vi "ReadJSONoverTCP.vi"(8 "error out":errorcluster, 11 "connection ID":refnum<k5>) -> (0 "error out":errorcluster, 2 "JSON":string, 3 "connection ID":refnum<k5>)   [LabVIEW 2018, in "feGEM DataPacker.lvlib"]
uses:
  feGEM DataPacker.lvlib
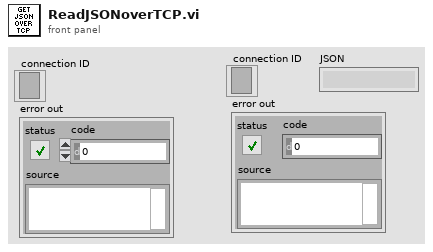
[diagram p1: front panel]
types:
  T1 = enum16{"Standard", "Buffered", "CRLF", "Immediate"}
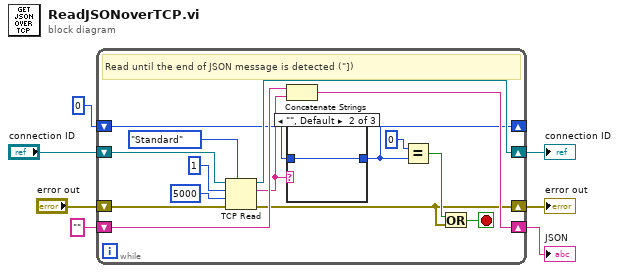
[diagram p0: block diagram]
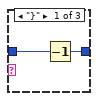
[diagram p2: hidden frame]
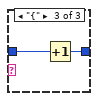
[diagram p3: hidden frame]
diagram:
  n1 = while {
    shift-right: [w21] -> w4
    shift-left: "connection ID" -> [w22]
    shift-right: [w12] -> w3
    shift-left: "error out" -> [w13]
    shift-right: [w19] -> w2
    shift-left: "" -> [w17]
    shift-right: [w9] -> _
    shift-left: 0 -> [w10]
    stop <- w15 stop-if-true
    # "Read until the end of JSON message is detected (\"])"
    n2 = TCP Read(connection ID=w22, bytes to read=1, error in (no error)=w13, 7:T1."Standard" ("mode (standard)"), 9:5000 ("timeout ms (25000)")) -> (connection ID out=w21:refnum<k5>, data out=w11:string, error out=w12:errorcluster)
    n3 = Concatenate Strings(w17, w11) -> (w19:string)
    n4 = case shown="\"\", Default" w11 {
      tunnel: w10 -> [w24 w25 w27]
      tunnel: [w23 w25 w26] -> w9
      frame "}" {
        n5 = Decrement(x=w24) -> (x-1=w23:i32)
      }
      frame "", Default {
      }
      frame "{" {
        n6 = Increment(x=w27) -> (x+1=w26:i32)
      }
    }
    n7 = Equal?(x=0, y=w9) -> (x = y?=w16:bool)
    n8 = Or(x=w16, y=w12) -> (x .or. y?=w15:bool)
  }
  "connection ID" <- w4
  "error out" <- w3
  "JSON" <- w2
